vi "Read Excel report.vi"(0 "report in":refnum<class "NI_Excel.lvclass">, 11 "error in (no error)":errorcluster) -> (4 "report out":refnum<class "NI_Excel.lvclass">, 8 "Excel report":T1, 15 "error out":errorcluster)   [LabVIEW 2017, in "NI_Excel.lvclass"]
uses:
  <vilib>/Utility/NIReport.llb/Excel/NI_Excel.lvclass
  <vilib>/Utility/NIReport.llb/Excel/NI_Excel.lvclass/NI_Excel.ctl
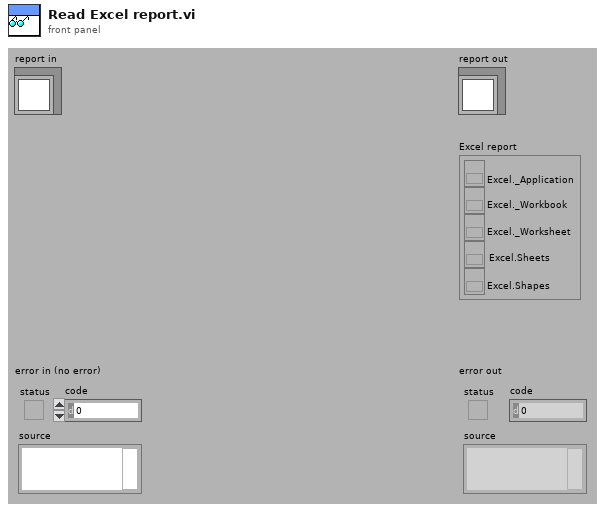
[diagram p1: front panel]
types:
  T1 = cluster{"Excel._Application":refnum<k7>, "Excel._Workbook":refnum<k7>, "Excel._Worksheet":refnum<k7>, "Excel.Sheets":refnum<k7>, "Excel.Shapes":refnum<k7>}
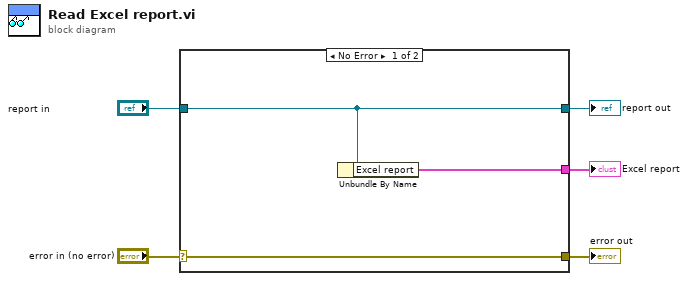
[diagram p0: block diagram]
diagram:
  n1 = case shown="No Error" "error in (no error)" {
    selector: "error in (no error)" -> [w8 w9]
    tunnel: [w8 w9] -> w4
    tunnel: [w7 w10] -> w2
    tunnel: "report in" -> [w7 w10]
    tunnel: [w6 _] -> w1
    frame No Error {
      n2 = Unbundle By Name(w7) -> ("Excel report"=w6:T1)
    }
    frame Error {
    }
  }
  "error out" <- w4
  "report out" <- w2
  "Excel report" <- w1
